vi "Server_solution.vi"() -> ()   [LabVIEW 2014]
uses:
  SubVIs/Server state.ctl
  SubVIs/Server data.ctl
  SubVIs/FGV action.ctl
panel:
  out "Action LED":bool
  out "IP":string
  out "Connection":bool
  out "Status display":string
  in  "stop":bool
  in  "port":u16
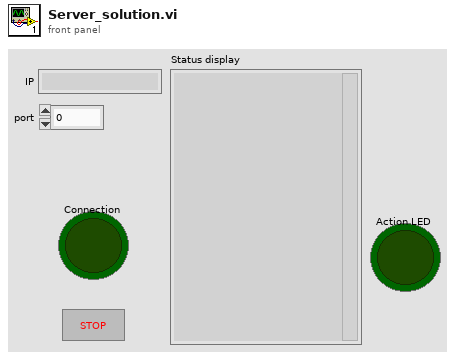
[diagram p1: front panel]
types:
  T1 = typedef "Server data.ctl" = cluster{"connection ID":refnum<k5>, "error IO":errorcluster, "Connection":bool}
  T2 = typedef "Server state.ctl" = enum16{"Init", "Listen", "Read", "Disconnect"}
  T3 = typedef "FGV action.ctl" = enum16{"Add", "Get", "Clear"}
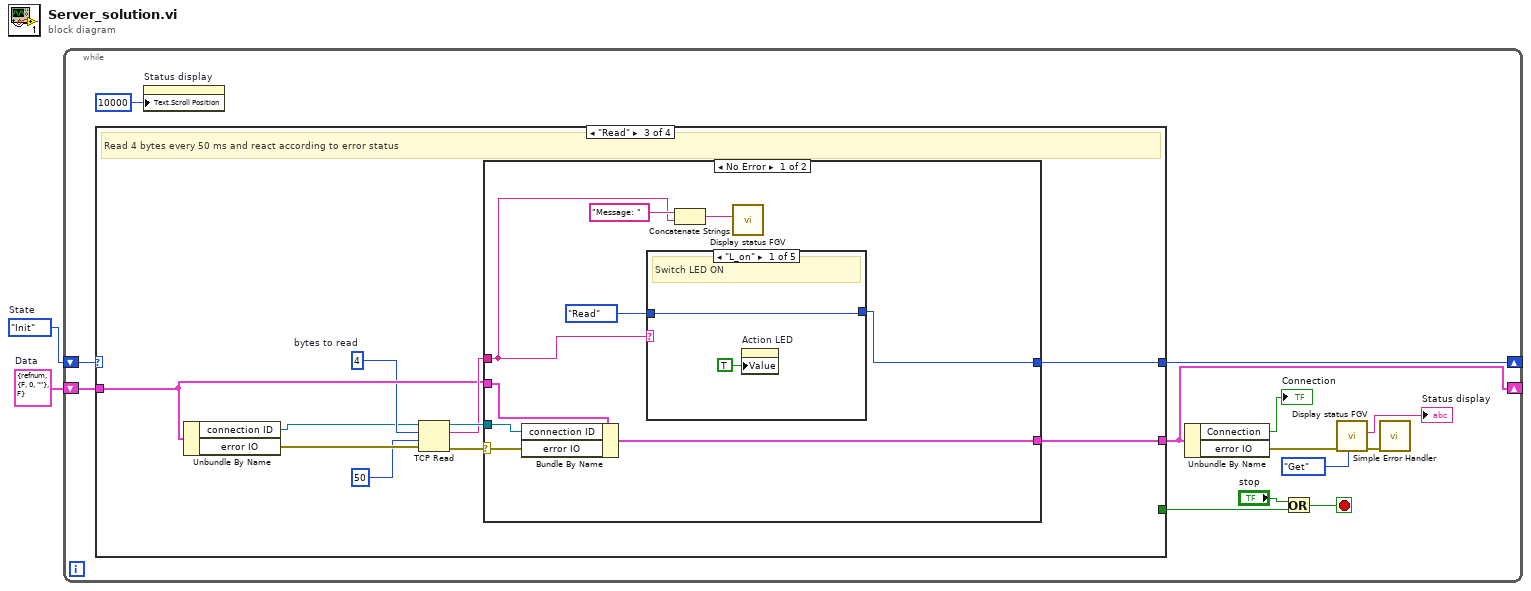
[diagram p0: block diagram]
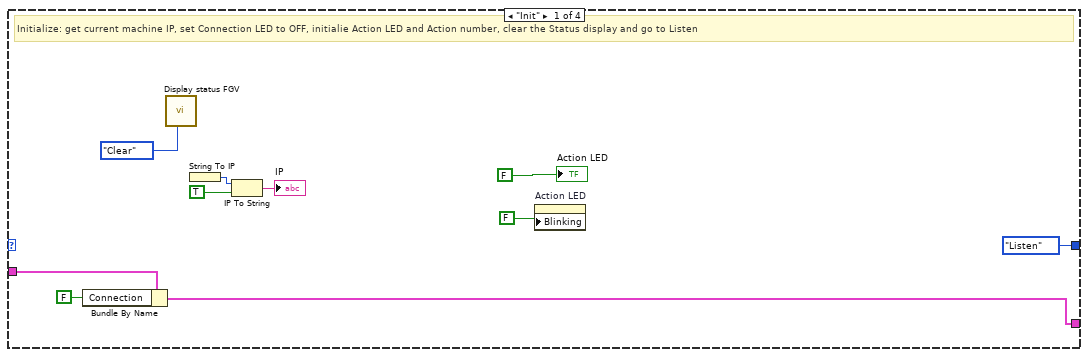
[diagram p2: hidden frame]
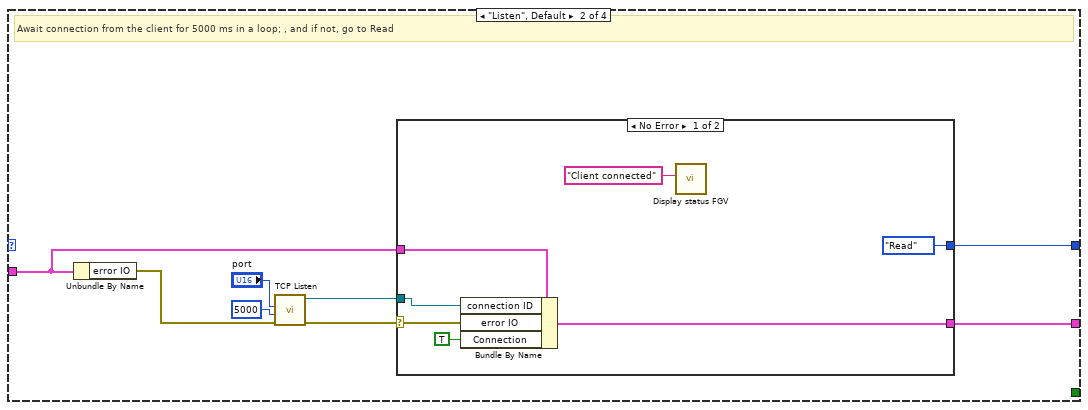
[diagram p3: hidden frame]
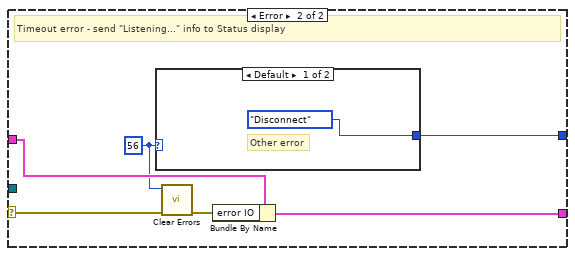
[diagram p4: hidden frame]
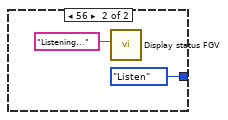
[diagram p5: hidden frame]
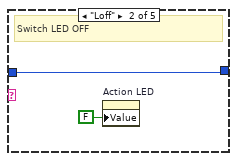
[diagram p6: hidden frame]
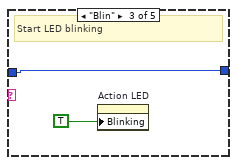
[diagram p7: hidden frame]
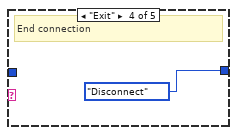
[diagram p8: hidden frame]
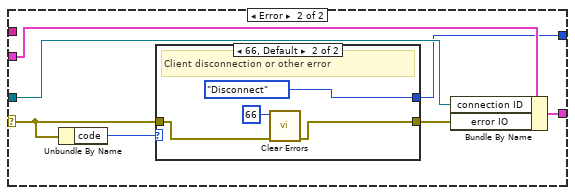
[diagram p10: hidden frame]
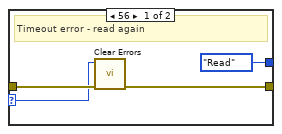
[diagram p11: hidden frame]
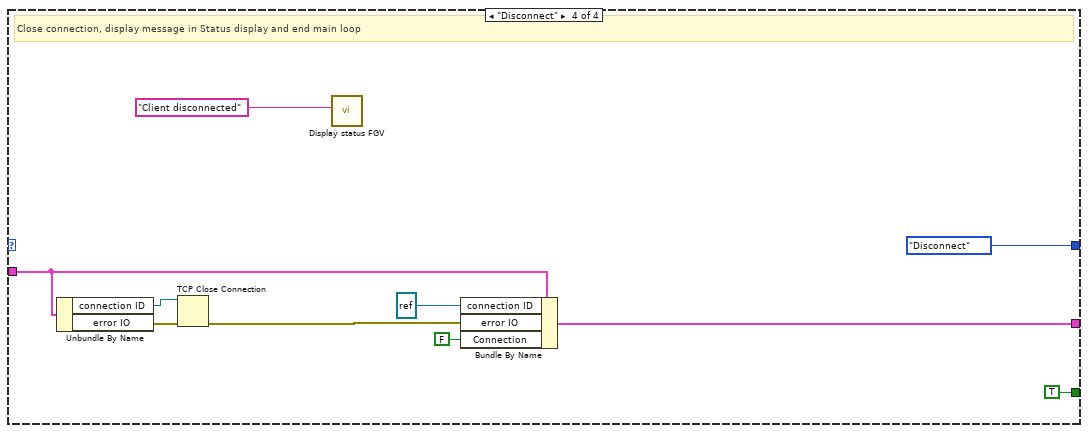
[diagram p12: hidden frame]
diagram:
  w1 = T1 {"connection ID"=refnum, "error IO"={"status"=FALSE, "code"=0, "source"=""}, "Connection"=FALSE}  # Data
  w2 = Server_state."Init"  # State
  n1 = while {
    shift-right: [w13] -> _
    shift-left: w2 -> [w15]
    shift-right: [w9] -> _
    shift-left: w1 -> [w14]
    stop <- w5 stop-if-true
    n2 = case shown="\"Read\"" w15 {
      tunnel: w14 -> [w25 w27 w56 w99]
      tunnel: [w24 w29 w54 w94] -> w9
      tunnel: [Server_state."Listen" ("Enum") w28 w52 Server_state."Disconnect" ("Enum")] -> w13
      tunnel: [_ _ _ TRUE ("stop")] -> w6
      frame "Init" {
        # "Initialize: get current machine IP, set Connection LED to OFF, initialie Action LED and Action number, clear the Status display and go to Listen"
        n3 = Bundle By Name(cluster=w25, "Connection"=FALSE) -> (w24:T1)
        n4 = call "Display status FGV.vi"("Action"=FGV_action."Clear") -> ()  [unwired: 9 in, 2 out]
        n5 = String To IP() -> (0:w20:u32)  [unwired: 1 in]
        n6 = IP To String(1:TRUE ("dot notation? (F)"), 2:w20) -> (0:→"IP":string)
        n7 = property on="Action LED" class="Bool (strict)"("Blinking"=FALSE ("Action LED")) -> ()  [unwired: 2 in, 2 out]
        "Action LED" <- FALSE ("Action LED")
      }
      frame "Listen", Default {
        # "Await connection from the client for 5000 ms in a loop; , and if not, go to Read"
        n8 = Unbundle By Name(w27) -> ("error IO"=w26:errorcluster)
        n9 = call <vilib>:"TCP Listen.vi"("error in (no error)"=w26, "timeout ms (wait forever: -1)"=5000, "port"="port") -> ("error out"=w31:errorcluster, "connection ID"=w30:refnum<k5>)  [unwired: 4 in, 3 out]
        n10 = case shown="No Error" w31 {
          selector: w31 -> [w35 w44]
          tunnel: w30 -> [w36 _]
          tunnel: w27 -> [w40 w46]
          tunnel: [w38 w45] -> w29
          tunnel: [Server_state."Read" ("Enum") w42] -> w28
          frame No Error {
            n11 = Bundle By Name(cluster=w40, "connection ID"=w36, "error IO"=w35, "Connection"=TRUE) -> (w38:T1)
            n12 = call "Display status FGV.vi"("Input"="Client connected" ("Status")) -> ()  [unwired: 9 in, 2 out]
          }
          frame Error {
            w43 = 56 ("specific error code to clear (0: all)")
            # "Timeout error - send \"Listening...\" info to Status display"
            n13 = case shown="Default" w43 {
              tunnel: [Server_state."Disconnect" ("Enum") Server_state."Listen" ("Enum")] -> w42
              frame Default {
                # "Other error"
              }
              frame 56 {
                n14 = call "Display status FGV.vi"("Input"="Listening..." ("Status")) -> ()  [unwired: 9 in, 2 out]
              }
            }
            n15 = call <vilib>:"Clear Errors.vi"("error in (no error)"=w44, "specific error code to clear (0: all)"=w43) -> ("error out"=w41:errorcluster)  [unwired: 4 in, 1 out]
            n16 = Bundle By Name(cluster=w46, "error IO"=w41) -> (w45:T1)
          }
        }
      }
      frame "Read" {
        w51 = 4  # bytes to read
        # "Read 4 bytes every 50 ms and react according to error status"
        n17 = Unbundle By Name(w56) -> ("connection ID"=w50:refnum<k5>, "error IO"=w59:errorcluster)
        n18 = TCP Read(connection ID=w50, bytes to read=w51, error in (no error)=w59, 9:50 ("timeout ms (25000)")) -> (connection ID out=w58:refnum<k5>, data out=w57:string, error out=w53:errorcluster)  [unwired: 1 in]
        n19 = case shown="No Error" w53 {
          selector: w53 -> [w66 w78]
          tunnel: w58 -> [w68 w83]
          tunnel: w57 -> [w62 _]
          tunnel: w56 -> [w65 w82]
          tunnel: [w67 w81] -> w54
          tunnel: [w60 w79] -> w52
          frame No Error {
            n20 = Bundle By Name(cluster=w65, "connection ID"=w68, "error IO"=w66) -> (w67:T1)
            n21 = case shown="\"L_on\"" w62 {
              tunnel: [w70 w72 w74 Server_state."Disconnect" ("Enum") w76] -> w60
              tunnel: Server_state."Read" ("Enum") -> [w70 w72 w74 _ w76]
              frame "L_on" {
                # "Switch LED ON"
                n22 = property on="Action LED" class="Bool (strict)"("Value"=TRUE ("Action LED")) -> ()  [unwired: 2 in, 2 out]
              }
              frame "Loff" {
                # "Switch LED OFF"
                n23 = property on="Action LED" class="Bool (strict)"("Value"=FALSE ("Action LED")) -> ()  [unwired: 2 in, 2 out]
              }
              frame "Blin" {
                # "Start LED blinking"
                n24 = property on="Action LED" class="Bool (strict)"("Blinking"=TRUE) -> ()  [unwired: 2 in, 2 out]
              }
              frame "Exit" {
                # "End connection"
              }
              frame Default {
                # "Do nothing"
              }
            }
            n25 = Concatenate Strings("Message: " ("string"), w62) -> (w63:string)
            n26 = call "Display status FGV.vi"("Input"=w63) -> ()  [unwired: 9 in, 2 out]
          }
          frame Error {
            n27 = Unbundle By Name(w78) -> ("code"=w80:i32)
            n28 = case shown="66, Default" w80 {
              selector: w80 -> [w84 _]
              tunnel: [Server_state."Read" ("Enum") Server_state."Disconnect" ("Enum")] -> w79
              tunnel: w78 -> [w86 w90]
              tunnel: [w85 w89] -> w77
              frame 56 {
                # "Timeout error - read again"
                n29 = call <vilib>:"Clear Errors.vi"("error in (no error)"=w86, "specific error code to clear (0: all)"=w84) -> ("error out"=w85:errorcluster)  [unwired: 4 in, 1 out]
              }
              frame 66, Default {
                # "Client disconnection or other error"
                n30 = call <vilib>:"Clear Errors.vi"("error in (no error)"=w90, "specific error code to clear (0: all)"=66) -> ("error out"=w89:errorcluster)  [unwired: 4 in, 1 out]
              }
            }
            n31 = Bundle By Name(cluster=w82, "connection ID"=w83, "error IO"=w77) -> (w81:T1)
          }
        }
      }
      frame "Disconnect" {
        # "Close connection, display message in Status display and end main loop"
        n32 = Unbundle By Name(w99) -> ("connection ID"=w101:refnum<k5>, "error IO"=w100:errorcluster)
        n33 = TCP Close Connection(connection ID=w101, error in (no error)=w100) -> (error out=w98:errorcluster)  [unwired: 1 in, 1 out]
        n34 = call "Display status FGV.vi"("Input"="Client disconnected" ("Status")) -> ()  [unwired: 9 in, 2 out]
        n35 = Bundle By Name(cluster=w99, "connection ID"=refnum<k5> refnum, "error IO"=w98, "Connection"=FALSE) -> (w94:T1)
      }
    }
    n36 = property on="Status display" class="Str"("Text.Scroll Position"=u32 10000) -> ()  [unwired: 2 in, 2 out]
    n37 = Unbundle By Name(w9) -> ("Connection"=→"Connection":bool, "error IO"=w4:errorcluster)
    n38 = Or(x="stop", y=w6) -> (x .or. y?=w5:bool)
    n39 = call "Display status FGV.vi"("Action"=FGV_action."Get", "error in"=w4) -> ("error out"=w3:errorcluster, "Display"=→"Status display":string)  [unwired: 8 in]
    n40 = call <vilib>:"Simple Error Handler.vi"("error in (no error)"=w3) -> ()  [unwired: 4 in, 5 out]
  }
